vi "Write_Log.vi"(3 "error in (no error)":errorcluster, 4 "Event data string":string, 5 "State":T1, 6 "dup path":path) -> (0 "error out":errorcluster)   [LabVIEW 2023]
doc: "Writes log file, takes array of values into spreadsheet .csv type of file"
uses:
  Controls/State.ctl
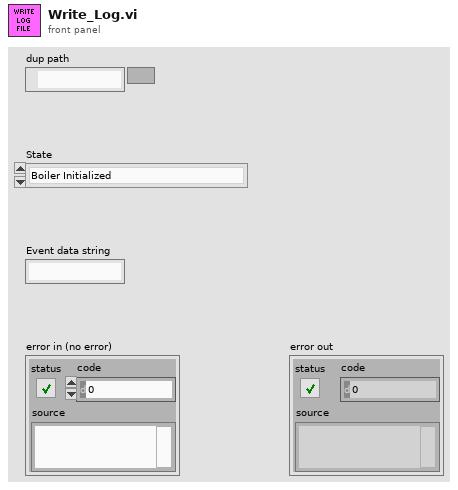
[diagram p1: front panel]
types:
  T1 = typedef "State.ctl" = enum16{"Boiler Initialized", "Boiler Ready", "Start Pre-Purge", "Pre-Purge Complete", "Pilot On", "Pilot Proved", "Force Draft Fan ON", "Boiler Running", "Start Shutdown Purge", "Shutdown Purge Complete", "Wait for Something"}
  T2 = enum16{"open", "replace", "create", "open or create", "replace or create", "replace or create with confirmation"}
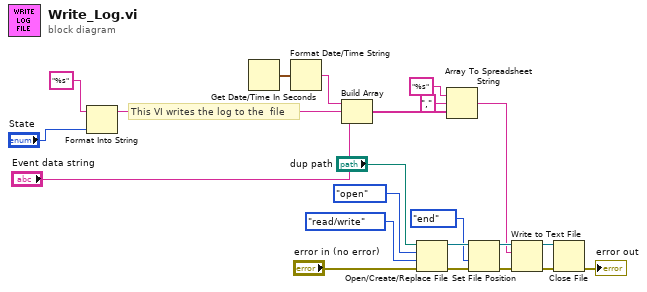
[diagram p0: block diagram]
diagram:
  # "This VI writes the log to the  file"
  n1 = Format Into String(format string="%s", "State") -> (resulting string=w3:string)  [unwired: 2 in, 1 out]
  n2 = Get Date/Time In Seconds() -> (seconds since 1Jan1904=w7:timestamp)
  n3 = Format Date/Time String(seconds (now)=w7) -> (date/time string=w5:string)  [unwired: 2 in]
  n4 = Build Array(w5, w3, "Event data string") -> (w6:string[])
  n5 = Open/Create/Replace File(file path (use dialog)="dup path", error in="error in (no error)", operation (0:open)=T2."open", access (0:read/write)=enum16{"read/write", "read-only", "write-only"}."read/write") -> (refnum out=w20:refnum<file>, error out=w21:errorcluster)  [unwired: 2 in, 1 out]
  n6 = Array To Spreadsheet String(delimiter (Tab)=",", array=w6, 3:"%s" ("format string")) -> (spreadsheet string=w18:string)
  n7 = Set File Position(refnum=w20, from (0:start)=enum16{"start", "end", "current"}."end", error in=w21) -> (refnum out=w22:refnum<file>, error out=w19:errorcluster)  [unwired: 1 in]
  n8 = Write to Text File(file (use dialog)=w22, text=w18, error in=w19) -> (refnum out=w11:refnum<file>, error out=w12:errorcluster)  [unwired: 1 in, 1 out]
  n9 = Close File(refnum=w11, error in=w12) -> (error out=→"error out":errorcluster)  [unwired: 1 out]
